vi "Load Display Settings.vi"(8 "error in (no error)":errorcluster, 11 "AF IMAQ Display in":refnum<class "HIJ Vision File Display.lvclass">) -> (0 "error out":errorcluster, 3 "AF IMAQ Display out":refnum<class "HIJ Vision File Display.lvclass">)   [LabVIEW 2014, in "HIJ Vision File Display.lvlib" / "HIJ Vision File Display.lvclass"]
uses:
  HIJ Vision File Display.lvclass
  Analyze/Analyze Parameter/Analyze Parameter Calibration/Analyze Parameter Calibration.lvclass
  HIJ Vision File Display.lvclass/HIJ Vision File Display.ctl
  HIJ Vision Display/HIJ Vision Display/HIJ Vision Display.lvclass/HIJ Vision Display.ctl
  Analyze/Analyze Parameter/Analyze Parameter Calibration/Analyze Parameter Calibration.lvclass/Analyze Parameter Calibration.ctl
  HIJ Vision Display/HIJ Vision Display/Read Display settings.vi
  HIJ Vision Display/HIJ Vision Display/Write Display settings.vi
  <vilib>/Utility/config.llb/Read Key (Double).vi
  HIJ Vision Display/HIJ Vision Display/HIJ Vision Display.lvclass
  <vilib>/Utility/config.llb/NI_LVConfig.lvlib
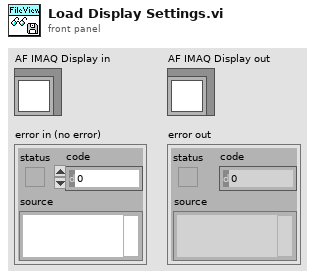
[diagram p1: front panel]
types:
  T1 = typedef "NI_LVConfig.lvlib/Config Data RefNum.ctl" = refnum<k1>
  T2 = typedef "DisplaySettings.ctl" = cluster{"Min. Thresh.":sgl, "X":dbl, "Y":dbl, "ShowLineout":bool, "ScaleParts":i32, "ShowLegende":bool, "Target Cross":bool, "Centroid Cross":bool, "Target color":u32, "Centroid color":u32, "calibr. µm/px":sgl[unit]}
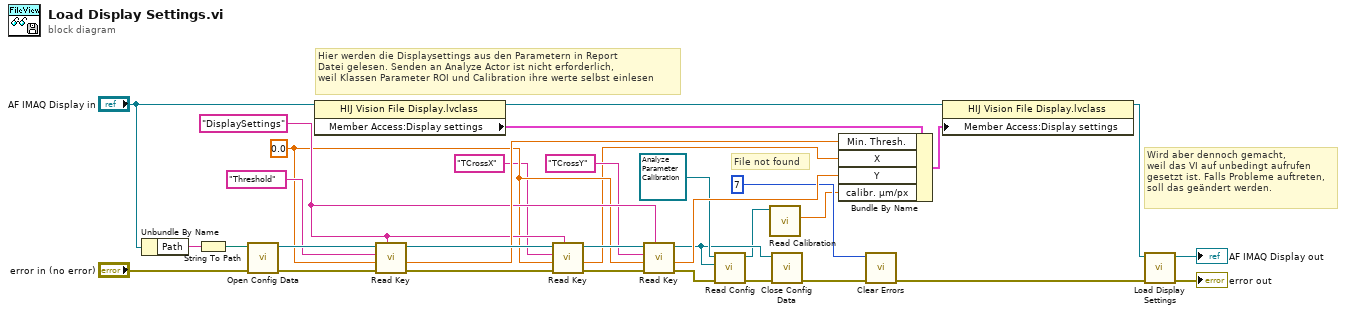
[diagram p0: block diagram]
diagram:
  w21 = 0.0
  w22 = "DisplaySettings" ("section")
  # "File not found"
  # "Wird aber dennoch gemacht,\nweil das VI auf unbedingt aufrufen\ngesetzt ist. Falls Probleme auftreten,\nsoll das geändert werden."
  # "Hier werden die Displaysettings aus den Parametern in Report \nDatei gelesen. Senden an Analyze Actor ist nicht erforderlich,\nweil Klassen Parameter ROI und Calibration ihre werte selbst einlesen"
  n1 = Unbundle By Name("AF IMAQ Display in") -> ("Path"=w33:string)
  n2 = String To Path(string=w33) -> (path=w32:path)
  n3 = call <vilib>:"Open Config Data.vi"("error in (no error)"="error in (no error)", "configuration file path"=w32) -> ("error out"=w26:errorcluster, "refnum"=w31:T1)  [unwired: 7 in, 1 out]
  n4 = property class="HIJ Vision File Display.lvclass"(reference="AF IMAQ Display in") -> (reference out=w14:refnum<class "HIJ Vision File Display.lvclass">, "Member Access:Display settings"=w13:T2)  [unwired: 1 in, 1 out]
  n5 = call-poly <vilib>:"Read Key.vi"("section"=w22, "error in (no error)"=w26, "default value"=w21, "key"="Threshold", "refnum"=w31) -> ("error out"=w29:errorcluster, "value"=w23:dbl, "refnum out"=w30:T1)  [unwired: 3 in, 1 out]
  n6 = call-poly <vilib>:"Read Key.vi"("section"=w22, "error in (no error)"=w29, "default value"=w21, "key"="TCrossX", "refnum"=w30) -> ("error out"=w27:errorcluster, "value"=w18:dbl, "refnum out"=w28:T1)  [unwired: 3 in, 1 out]
  n7 = call-poly <vilib>:"Read Key.vi"("section"=w22, "error in (no error)"=w27, "default value"=w21, "key"="TCrossY", "refnum"=w28) -> ("error out"=w4:errorcluster, "value"=w17:dbl, "refnum out"=w5:T1)  [unwired: 3 in, 1 out]
  n8 = call-dynamic "Read Config.vi"("error in (no error)"=w4, "Resource In"=w5, "Analyze Parameter Calibration in"=refnum<class "Analyze Parameter Calibration.lvclass"> refnum ("Analyze Parameter Calibration.lvclass")) -> ("error out"=w3:errorcluster, "Analyze Parameter Calibration out"=w2:refnum<class "Analyze Parameter Calibration.lvclass">)  [unwired: 6 in, 1 out]
  n9 = call "Read Calibration.vi"("Analyze Parameter Calibration in"=w2) -> ("Calibration"=w1:dbl[unit])  [unwired: 8 in, 2 out]
  n10 = call <vilib>:"Close Config Data.vi"("error in (no error)"=w3, "refnum"=w5) -> ("error out"=w10:errorcluster)  [unwired: 8 in, 1 out]
  n11 = Bundle By Name(cluster=w13, "Min. Thresh."=w23, "X"=w18, "Y"=w17, "calibr. µm/px"=w1) -> (w24:T2)
  n12 = call <vilib>:"Clear Errors.vi"("error in (no error)"=w10, "specific error code to clear (0: all)"=7) -> ("error out"=w8:errorcluster)  [unwired: 4 in, 1 out]
  n13 = property class="HIJ Vision File Display.lvclass"(reference=w14, "Member Access:Display settings"=w24) -> (reference out=w12:refnum<class "HIJ Vision File Display.lvclass">)  [unwired: 1 in, 1 out]
  n14 = call-parent "Load Display Settings.vi"("error in (no error)"=w8, "AF IMAQ Display in"=w12) -> ("error out"=→"error out":errorcluster, "AF IMAQ Display out"=→"AF IMAQ Display out":refnum<class "HIJ Vision File Display.lvclass">)  [unwired: 8 in]
